vi "BeadScannerHost.vi"() -> ()   [LabVIEW 2016]
uses:
  <vilib>/Utility/file.llb/Write Delimited Spreadsheet (string).vi
  <vilib>/Analysis/3filter.llb/Butterworth Filter (DBL).vi
  <vilib>/Utility/file.llb/Write Delimited Spreadsheet (DBL).vi
  <vilib>/gmath/NI_Gmath.lvlib
  <vilib>/Analysis/NI_AALBase.lvlib
panel:
  out "Shutter Open":bool
  out "Stored!":bool
  in  "Select Bead":u16(ring) items=["Center #1", "Robot #2", "Window #3"]
  in  "Store Bead For Triggers":bool
  out "size(s) 3":i32
  out "size(s) 2":i32
  out "size(s)":i32
  in  "Max Wire Feed Adjustment":dbl=1.5
  in  "mm/sample":dbl=0.5 format="%#_13g"
  in  "Write Robot Correction":bool=TRUE
  out "Waveform Graph 2":waveform(dbl)(graph)={"t0"=timestamp(0 s since 1904-01-01), "dt"=1.0, "Y"=[0.0, 0.0, 0.0, 0.0, 0.0, 0.0, 0.0, 0.0, 0.0, 0.0, 0.0, 0.0, 0.0, 0.0, 0.0, 0.0, 0.0, 0.0, 0.0, 0.0, 0.0, 0.0, 0.0, 0.0, 0.0, 0.0, 0.0, 0.0, 0.0, 0.0, 0.0, 0.0, 0.0, 0.0, 0.0, 0.0, 0.0, 0.0, 0.0, 0.0, 0.0, 0.0, 0.0, 0.0, 0.0, 0.0, 0.0, 0.0, 0.0, 0.0, 0.0, 0.0, 0.0, 0.0, 0.0, 0.0, 0.0, 0.0, 0.0, 0.0, 0.0, 0.0, 0.0, 0.0, 0.0, 0.0, 0.0, 0.0, 0.0, 0.0, 0.0, 0.0, 0.0, 0.0, 0.0, 0.0, 0.0, 0.0, 0.0, 0.0, 0.0, 0.0, 0.0, 0.0, 0.0, 0.0, 0.0, 0.0, 0.0, 0.0, 0.0, 0.0, 0.0, 0.0, 0.0, 0.0, 0.0, 0.0, 0.0, 0.0, 0.0, 0.0, 0.0, 0.0, 0.0, 0.0, 0.0, 0.0, 0.0, 0.0, 0.0, 0.0, 0.0, 0.0, 0.0, 0.0, 0.0, 0.0, 0.0, 0.0, 0.0, 0.0, 0.0, 0.0, 0.0, 0.0, 0.0, 0.0, 0.0, 0.0, 0.0, 0.0, 0.0, 0.0, 0.0, 0.0, 0.0, 0.0, 0.0, 0.0, 0.0, 0.0, 0.0, 0.0, 0.0, 0.0, 0.0, 0.0, 0.0, 0.0, 0.0, 0.0, 0.0, 0.0, 0.0, 0.0, 0.0, 0.0, 0.0, 0.0, 0.0, 0.0, 0.0, 0.0, 0.0, 0.0, 0.0, 0.0, 0.0, 0.0, 0.0, 0.0, 0.0, 0.0, 0.0, 0.0, 0.0, 0.0, 0.0, 0.0, 0.0, 0.0, 0.0, 0.0, 0.0, 0.0, 0.0, 0.0, 0.0, 0.0, 0.0, 0.0, 0.0, 0.0, 0.0, 0.0, 0.0, 0.0, 0.0, 0.0, 0.0, 0.0, 0.0, 0.0, 0.0, 0.0, 0.0, 0.0, 0.0, 0.0, 0.0, 0.0, 0.0, 0.0, 0.0, 0.0, 0.0, 0.0, 0.0, 0.0, 0.0, 0.0, 0.0, 0.0, 0.0, 0.0, 0.0, 0.0, 0.0, 0.0, 0.0, 0.0, 0.0, 0.0, 0.0, 0.0, 0.0, 0.0, 0.0, 0.0, 0.0, 0.0, 0.0, 0.0, 0.0, 0.0, 0.0, 0.0, 0.0, 0.0, 0.0, 0.0, 0.0, 0.0, 0.0, 0.0, 0.0, 0.0, 0.0, 0.0, 0.0, 0.0, 0.0, 0.0, 0.0, 0.0, 0.0, 0.0, 0.0, 0.0, 0.0, 0.0, 0.0, 0.0, 0.0, 0.0, 0.0, 0.0, 0.0, 0.0, 0.0, 0.0, 0.0, 0.0, 0.0, 0.0, 0.0, 0.0, 0.0, 0.0, 0.0, 0.0, 0.0, 0.0, 0.0, 0.0, 0.0, 0.0, 0.0, 0.0, 0.0, 0.0, 0.0, 0.0, 0.0, 0.0, 0.0, 0.0, 0.0, 0.0, 0.0, 0.0, 0.0, 0.0, 0.0, 0.0, 0.0, 0.0, 0.0, 0.0, 0.0, 0.0, 0.0, 0.0, 0.0, 0.0, 0.0, 0.0, 0.0, 0.0, 0.0, 0.0, 0.0, 0.0, 0.0, 0.0, 0.0, 0.0, 0.0, 0.0, 0.0, 0.0, 0.0, 0.0, 0.0, 0.0, 0.0, 0.0, 0.0, 0.0, 0.0, 0.0, 0.0, 0.0, 0.0, 0.0, 0.0, 0.0, 0.0, 0.0, 0.0, 0.0, 0.0, 0.0, 0.0, 0.0, 0.0, 0.0, 0.0, 0.0, 0.0, 0.0, 0.0, 0.0, 0.0, 0.0, 0.0, 0.0, 0.0, 0.0, 0.0, 0.0, 0.0, 0.0, 0.0, 0.0, 0.0, 0.0, 0.0, 0.0, 0.0, 0.0, 0.0, 0.0, 0.0, 0.0, 0.0, 0.0, 0.0, 0.0, 0.0, 0.0, 0.0, 0.0, 0.0, 0.0, 0.0, 0.0, 0.0, 0.0, 0.0, 0.0, 0.0, 0.0, 0.0, 0.0, 0.0, 0.0, 0.0, 0.0, 0.0, 0.0, 0.0, 0.0, 0.0, 0.0, 0.0, 0.0, 0.0, 0.0, 0.0, 0.0, 0.0, 0.0, 0.0, 0.0, 0.0, 0.0, 0.0, 0.0, 0.0, 0.0, 0.0, 0.0, 0.0, 0.0, 0.0, 0.0, 0.0, 0.0, 0.0, 0.0, 0.0, 0.0, 0.0, 0.0, 0.0, 0.0, 0.0, 0.0, 0.0, 0.0, 0.0, 0.0, 0.0, 0.0, 0.0, 0.0, 0.0, 0.0, 0.0, 0.0, 0.0, 0.0, 0.0, 0.0, 0.0, 0.0, 0.0, 0.0, 0.0, 0.0]}
  out "Waveform Graph":waveform(dbl)(graph)={"t0"=timestamp(0 s since 1904-01-01), "dt"=1.0, "Y"=array[482 elements]}
  in  "Deadband":dbl=0.1
  in  "Override Gain":dbl=1.0 format="%#_13g"
  in  "Programmed Layer Height (mm)":dbl=1.5 format="%#_13g"
  in  "Laser Bias (mm)":dbl=10.0 format="%#_13g"
  in  "base path":path=path "C:/Users/Mark/Desktop/BeadScan"
  out "Bead Number":i32=1
  in  "stop":bool
  # "laser bias history\n-62.0272"
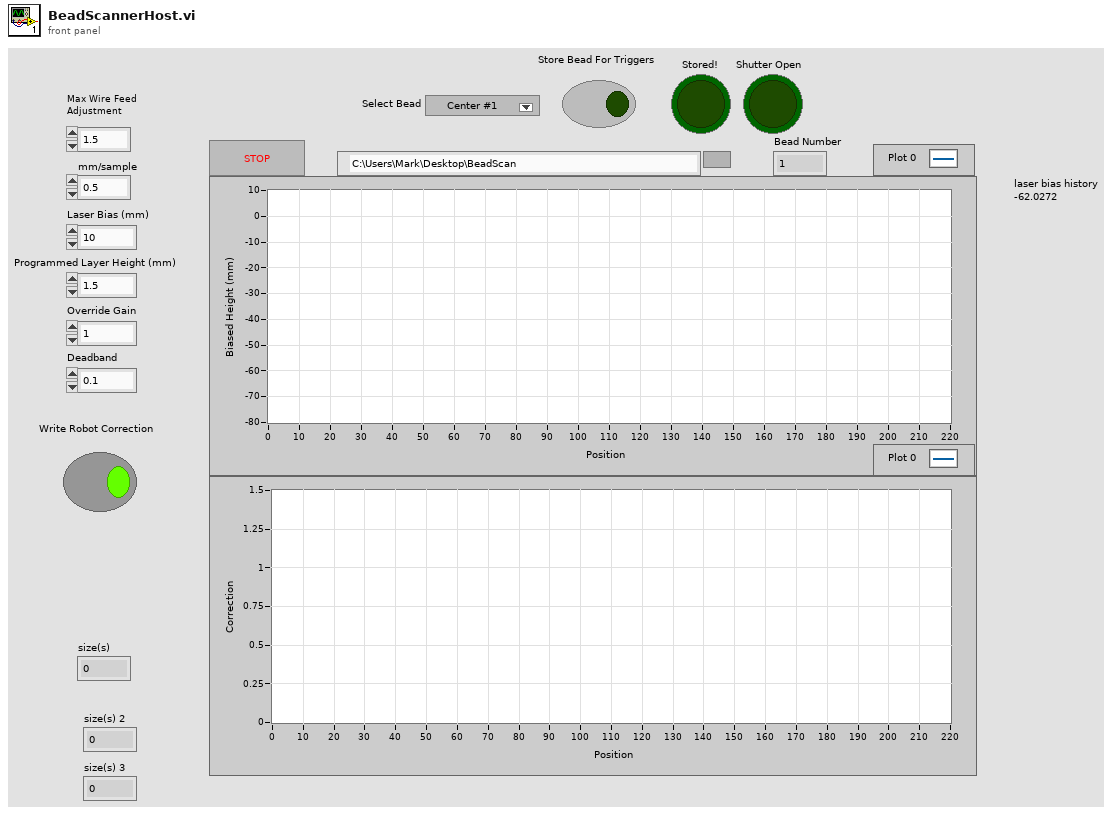
[diagram p1: front panel]
types:
  T1 = enum16{"open", "replace", "create", "open or create", "replace or create", "replace or create with confirmation"}
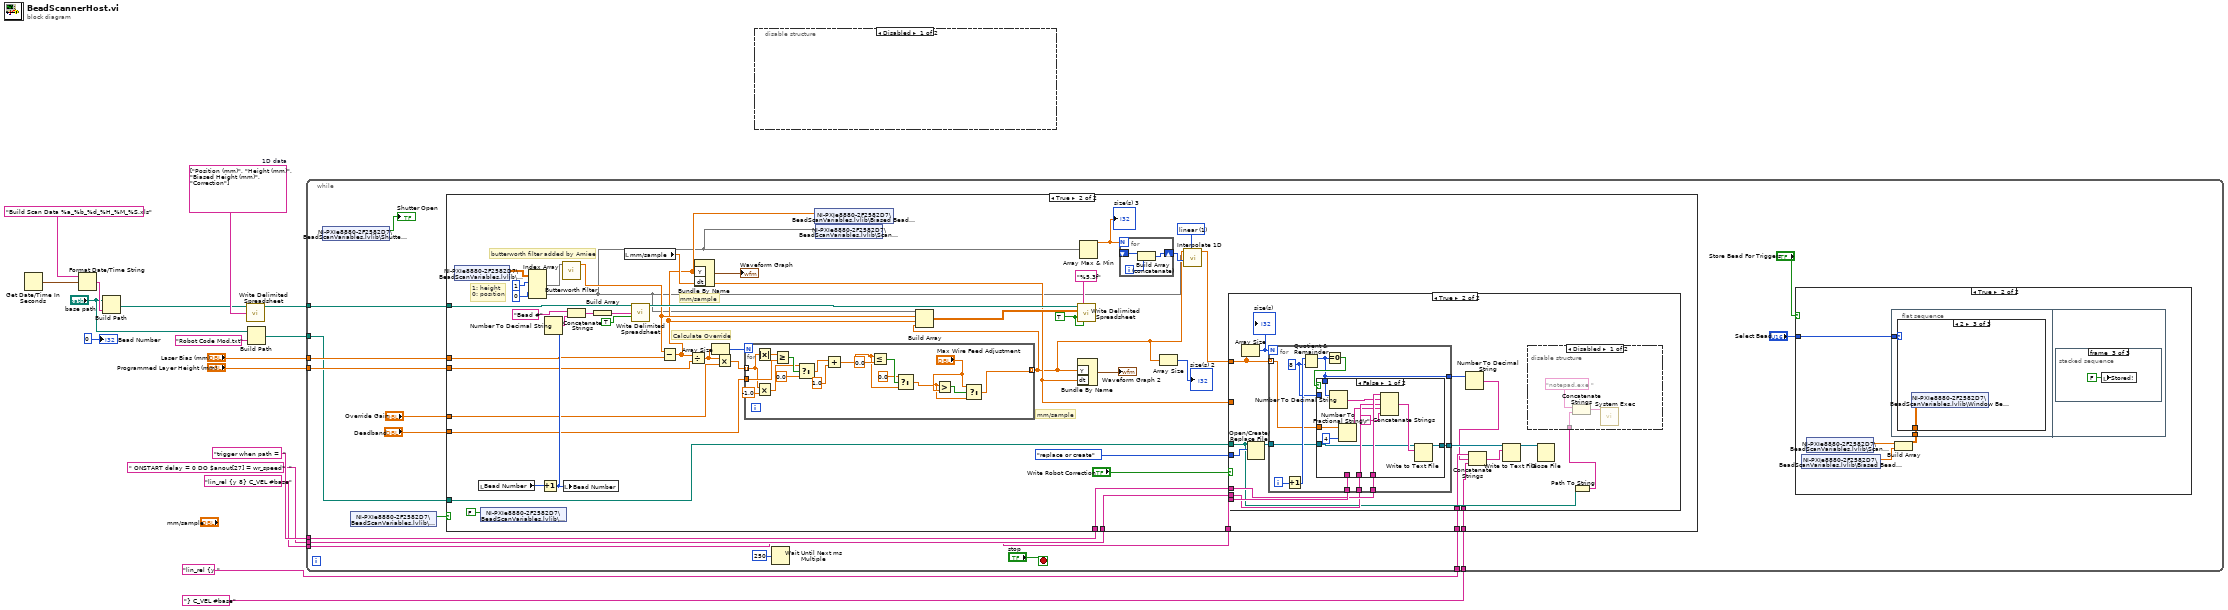
[diagram p0: block diagram]
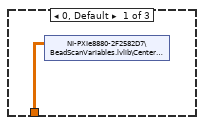
[diagram p4: hidden frame]
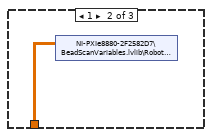
[diagram p5: hidden frame]
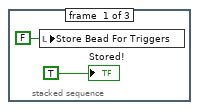
[diagram p6: hidden frame]
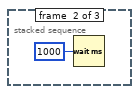
[diagram p7: hidden frame]
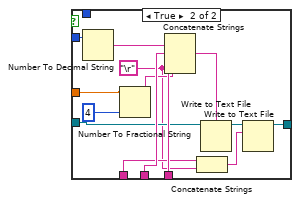
[diagram p11: hidden frame]
diagram:
  w13 = string[] ["Position (mm)", "Height (mm)", "Biased Height (mm)", "Correction"]  # 1D data
  n1 = Get Date/Time In Seconds() -> (seconds since 1Jan1904=w17:timestamp)
  n2 = Format Date/Time String(time format string (%c)="Build Scan Data %a_%b_%d_%H_%M_%S.xls", seconds (now)=w17) -> (date/time string=w15:string)  [unwired: 1 in]
  n3 = Build Path(base path="base path", name or relative path=w15) -> (appended path=w12:path)
  n4 = call-poly <vilib>:"Write Delimited Spreadsheet.vi"("file path (dialog if empty)"=w12, "1D data"=w13) -> ("new file path (Not A Path if cancelled)"=w11:path)  [unwired: 12 in, 1 out]
  n5 = Build Path(base path="base path", name or relative path="Robot Code Mod.txt") -> (appended path=w6:path)
  n6 = while {
    tunnel: w11 -> [w31]
    tunnel: "Laser Bias (mm)" -> [w30]
    tunnel: "Programmed Layer Height (mm)" -> [w29]
    tunnel: w6 -> [w26]
    tunnel: "trigger when path =  " -> [w25]
    tunnel: " ONSTART delay = 0 DO $anout[27] = wr_speed*  " -> [w24]
    tunnel: "lin_rel {y 8} C_VEL #base" -> [w23]
    tunnel: "lin_rel {y " -> [w22]
    tunnel: "} C_VEL #base" -> [w21]
    stop <- "stop" stop-if-true
    n7 = shared-variable "NI-PXIe8880-2F2582D7\\BeadScanVariables.lvlib\\Shutter Open"() -> (→"Shutter Open":bool)  [unwired: 1 in, 1 out]
    n8 = shared-variable "NI-PXIe8880-2F2582D7\\BeadScanVariables.lvlib\\BeadScanComplete"() -> (w32:bool)  [unwired: 1 in, 1 out]
    n9 = case shown="True" w32 {
      tunnel: w31 -> [_ w82]
      tunnel: w30 -> [_ w77]
      tunnel: w29 -> [_ w76]
      tunnel: "Override Gain" -> [_ w75]
      tunnel: "Deadband" -> [_ w71]
      tunnel: w26 -> [_ w65]
      tunnel: w25 -> [_ w63]
      tunnel: w24 -> [_ w62]
      tunnel: w23 -> [_ w61]
      tunnel: w22 -> [_ w60]
      tunnel: w21 -> [_ w59]
      frame False {
      }
      frame True {
        w57 = 1 items=["nearest", "linear", "spline", "cubic Hermite", "Lagrange"] ("method")
        w90 = TRUE ("append to file? (new file:F)")
        # "butterworth filter added by Amiee"
        # "1: height\n0: position"
        # "mm/sample"
        # "mm/sample"
        # "Calculate Override"
        n10 = shared-variable "NI-PXIe8880-2F2582D7\\BeadScanVariables.lvlib\\ScanData"() -> (w79:dbl[][])  [unwired: 1 in, 1 out]
        n11 = local read "Bead Number"() -> (w88:i32)
        n12 = shared-variable "NI-PXIe8880-2F2582D7\\BeadScanVariables.lvlib\\BeadScanComplete"(FALSE ("BeadScanComplete")) -> ()  [unwired: 1 in, 1 out]
        n13 = Index Array(array=w79, index (row) #1=1 ("index (row)"), index (row) #2=0 ("index (row)")) -> (element #1=w51:dbl[], element #2=w48:dbl[])  [unwired: 2 in]
        n14 = Increment(x=w88) -> (x+1=w86:i32)
        n15 = Number To Decimal String(number=w86) -> (decimal integer string=w85:string)  [unwired: 1 in]
        n16 = call-poly <vilib>:"Butterworth Filter.vi"("X"=w51) -> ("Filtered X"=w50:dbl[])  [unwired: 7 in, 1 out]
        n17 = local write "Bead Number"(w86) -> ()
        n18 = Concatenate Strings("Bead #", w85) -> (w84:string)
        n19 = Build Array(w84) -> (w83:string[])
        n20 = local read "mm/sample"() -> (w66:dbl)
        n21 = call-poly <vilib>:"Write Delimited Spreadsheet.vi"("file path (dialog if empty)"=w82, "1D data"=w83, "append to file? (new file:F)"=TRUE) -> ("new file path (Not A Path if cancelled)"=w81:path)  [unwired: 11 in, 1 out]
        n22 = Subtract(x=w50, y=w77) -> (x-y=w49:dbl[])
        n23 = Divide(x=w49, y=w76) -> (x/y=w73:dbl[])
        n24 = Bundle By Name("Y"=w49, "dt"=w66) -> (→"Waveform Graph":waveform(dbl))  [unwired: 1 in]
        n25 = Array Size(array=w73) -> (size(s)=w74:i32)
        n26 = Multiply(x=w73, y=w75) -> (x*y=w72:dbl[])
        n27 = for {
          N: w74 -> [_]
          tunnel: w72 -> [w156] mode=indexing
          tunnel: w71 -> [w165]
          tunnel: [w150] -> w55 mode=indexing
          n28 = Absolute Value(x=w156) -> (abs(x)=w166:dbl)
          n29 = Multiply(x=w156, y=-1.0) -> (x*y=w154:dbl)
          n30 = Greater Or Equal?(x=w166, y=w165) -> (x >= y?=w164:bool)
          n31 = Select(t=w154, s=w164, f=0.0) -> (s? t:f=w158:dbl)
          n32 = Add(x=w158, y=1.0) -> (x+y=w157:dbl)
          n33 = Less Or Equal?(x=w157, y=0.0) -> (x <= y?=w162:bool)
          n34 = Select(t=0.0, s=w162, f=w157) -> (s? t:f=w151:dbl)
          n35 = Greater?(x=w151, y="Max Wire Feed Adjustment") -> (0:w153:bool)
          n36 = Select(t="Max Wire Feed Adjustment", s=w153, f=w151) -> (s? t:f=w150:dbl)
        }
        n37 = shared-variable "NI-PXIe8880-2F2582D7\\BeadScanVariables.lvlib\\Biased Bead Scan"(w49) -> ()  [unwired: 1 in, 1 out]
        n38 = shared-variable "NI-PXIe8880-2F2582D7\\BeadScanVariables.lvlib\\Scan Position"(w48) -> ()  [unwired: 1 in, 1 out]
        n39 = Build Array(w48, w50, w49, w55) -> (w69:dbl[][])
        n40 = call-poly <vilib>:"Write Delimited Spreadsheet.vi"("file path (dialog if empty)"=w81, "format (%.3f)"="%5.3f", "2D data"=w69, "append to file? (new file:F)"=w90, "transpose? (no:F)"=w90) -> ()  [unwired: 9 in, 2 out]
        n41 = Bundle By Name("Y"=w55, "dt"=w66) -> (→"Waveform Graph 2":waveform(dbl))  [unwired: 1 in]
        n42 = Array Max & Min(array=w48) -> (max value=w53:dbl)  [unwired: 3 out]
        "size(s) 3" <- w53
        n43 = for {
          N: w53 -> [_]
          shift-right: [w92] -> w56
          shift-left: _ -> [w94]
          i -> [w93]
          n44 = Build Array (concatenate)(w94, w93) -> (w92:i32[])
        }
        n45 = Array Size(array=w55) -> (size(s)=→"size(s) 2":i32)
        n46 = call <vilib>:"Interpolate 1D.vi"("method"=w57, "xi"=w56, "X"=w48, "Y"=w55) -> ("yi"=w52:dbl[])  [unwired: 5 in, 2 out]
        n47 = case shown="True" "Write Robot Correction" {
          tunnel: w52 -> [_ w109]
          tunnel: w66 -> [_ _]
          tunnel: w65 -> [_ w103]
          tunnel: T1."replace or create" ("operation (0:open)") -> [_ w108]
          tunnel: w63 -> [_ w105]
          tunnel: w62 -> [_ w104]
          tunnel: w61 -> [_ w106]
          tunnel: w60 -> [_ w98]
          tunnel: w59 -> [_ w97]
          frame False {
          }
          frame True {
            n48 = Array Size(array=w109) -> (size(s)=w110:i32)
            "size(s)" <- w110
            n49 = Open/Create/Replace File(file path (use dialog)=w103, operation (0:open)=w108) -> (refnum out=w107:refnum<file>)  [unwired: 4 in, 2 out]
            n50 = for {
              N: w110 -> [_]
              tunnel: w109 -> [w117] mode=indexing
              tunnel: w107 -> [w121]
              tunnel: w106 -> [w120]
              tunnel: w105 -> [w119]
              tunnel: w104 -> [w118]
              tunnel: [w116] -> w101
              tunnel: [w114] -> w96
              i -> [w124]
              w115 = 8 ("y")
              n51 = Increment(x=w124) -> (x+1=w123:i32)
              n52 = Quotient & Remainder(x=w123, y=w115) -> (x-y*floor(x/y)=w114:i32)  [unwired: 1 out]
              n53 = Equal To 0?(x=w114) -> (x = 0?=w122:bool)
              n54 = case shown="False" w122 {
                tunnel: w121 -> [w127 w142]
                tunnel: w120 -> [_ w139]
                tunnel: w114 -> [w135 _]
                tunnel: w119 -> [w134 w149]
                tunnel: w118 -> [w130 w145]
                tunnel: w117 -> [w132 w147]
                tunnel: [w126 w141] -> w116
                tunnel: w115 -> [_ w136]
                frame False {
                  n55 = Number To Decimal String(number=w135) -> (decimal integer string=w133:string)  [unwired: 1 in]
                  n56 = Number To Fractional String(number=w132, precision (6)=i16 4) -> (F-format string=w129:string)  [unwired: 2 in]
                  n57 = Concatenate Strings(w134, w133, w130, w129, "\r") -> (w128:string)
                  n58 = Write to Text File(file (use dialog)=w127, text=w128) -> (refnum out=w126:refnum<file>)  [unwired: 2 in, 2 out]
                }
                frame True {
                  w138 = "\r"
                  n59 = Number To Decimal String(number=w136) -> (decimal integer string=w148:string)  [unwired: 1 in]
                  n60 = Number To Fractional String(number=w147, precision (6)=i16 4) -> (F-format string=w144:string)  [unwired: 2 in]
                  n61 = Concatenate Strings(w149, w148, w145, w144, w138) -> (w143:string)
                  n62 = Concatenate Strings(w139, w138) -> (w137:string)
                  n63 = Write to Text File(file (use dialog)=w142, text=w143) -> (refnum out=w140:refnum<file>)  [unwired: 2 in, 2 out]
                  n64 = Write to Text File(file (use dialog)=w140, text=w137) -> (refnum out=w141:refnum<file>)  [unwired: 2 in, 2 out]
                }
              }
            }
            n65 = Number To Decimal String(number=w96) -> (decimal integer string=w95:string)  [unwired: 1 in]
            n66 = Concatenate Strings(w98, w95, w97) -> (w99:string)
            n67 = Write to Text File(file (use dialog)=w101, text=w99) -> (refnum out=w100:refnum<file>)  [unwired: 2 in, 2 out]
            n68 = Close File(refnum=w100) -> ()  [unwired: 1 in, 2 out]
            n69 = Path To String(path=w103) -> (string=w102:string)
            n70 = disable-structure shown="Disabled" {
              disable-tunnel: w102 -> [w112 _]
              frame Disabled {
                n71 = Concatenate Strings("notepad.exe " ("command line"), w112) -> (w111:string)
                n72 = call <vilib>:"System Exec.vi"("command line"=w111) -> ()  [unwired: 7 in, 4 out]
              }
              frame Enabled {
              }
            }
          }
        }
      }
    }
    n73 = Wait Until Next ms Multiple(millisecond multiple=u32 250) -> ()  [unwired: 1 out]
    n74 = case shown="True" "Store Bead For Triggers" {
      tunnel: "Select Bead" -> [_ w38]
      frame False {
      }
      frame True {
        n75 = shared-variable "NI-PXIe8880-2F2582D7\\BeadScanVariables.lvlib\\Biased Bead Scan"() -> (w36:dbl[])  [unwired: 1 in, 1 out]
        n76 = shared-variable "NI-PXIe8880-2F2582D7\\BeadScanVariables.lvlib\\Scan Position"() -> (w37:dbl[])  [unwired: 1 in, 1 out]
        n77 = flat-sequence {
          tunnel: w38 -> [w40]
          tunnel: w35 -> [w39]
          frame #0 {
            n78 = case shown="2" w40 {
              tunnel: w39 -> [w41 w42 w43]
              frame 0, Default {
                n79 = shared-variable "NI-PXIe8880-2F2582D7\\BeadScanVariables.lvlib\\Center Bead #1"(w41) -> ()  [unwired: 1 in, 1 out]
              }
              frame 1 {
                n80 = shared-variable "NI-PXIe8880-2F2582D7\\BeadScanVariables.lvlib\\Robot Bead #2"(w42) -> ()  [unwired: 1 in, 1 out]
              }
              frame 2 {
                n81 = shared-variable "NI-PXIe8880-2F2582D7\\BeadScanVariables.lvlib\\Window Bead #3"(w43) -> ()  [unwired: 1 in, 1 out]
              }
            }
          }
          frame #1 {
            n82 = stacked-sequence {
              frame #0 {
                n83 = local write "Store Bead For Triggers"(FALSE ("Store Bead For Triggers")) -> ()
                "Stored!" <- TRUE
              }
              frame #1 {
                n84 = Wait (ms)(milliseconds to wait=u32 1000) -> ()  [unwired: 1 out]
              }
              frame #2 {
                n85 = local write "Stored!"(FALSE ("Stored!")) -> ()
              }
            }
          }
        }
        n86 = Build Array(w37, w36) -> (w35:dbl[][])
      }
    }
  }
  n87 = disable-structure shown="Disabled" {
    frame Disabled {
    }
    frame Enabled {
    }
  }
  "Bead Number" <- 0 ("Bead Number")
